vi "ReadSensors.vi"(8 "error in":errorcluster, 11 "UART in":refnum<visa-resource-name>) -> (0 "error out":errorcluster, 2 "Kobuki Sensors  out":T1 {"Charger Source" items=["DISCHARGING"=0, "DOCKING_CHARGED"=2, "DOCKING_CHARGING"=6, "ADAPTER_CHARGED"=18, "ADAPTER_CHARGING"=22]}, 3 "UART out":refnum<visa-resource-name>)   [LabVIEW 2017]
uses:
  KobukiSensors.ctl
  Kobuki Bumps and WheelDrops.ctl
  Kobuki Buttons.ctl
  GetSensorState.ctl
  <vilib>/Instr/_visa.llb/VISA Flush IO Buffer Mask.ctl
  <vilib>/Utility/error.llb/Error Cluster From Error Code.vi
  <vilib>/ErrorRing/Error Ring.xnode
  system/RobotType.ctl
panel:
  out "raw gyro Z":u16(graph)
  out "raw gyro Y":u16(graph)
  out "raw gyro X":u16(graph)
  out "Array":u8[](array[numeric])
  out "Kobuki Sensors 3":T1 {"Charger Source" items=["DISCHARGING"=0, "DOCKING_CHARGED"=2, "DOCKING_CHARGING"=6, "ADAPTER_CHARGED"=18, "ADAPTER_CHARGING"=22]}
  out "Raw Sensors Value 3":u8[][](array[numeric])=[[1, 15, 200, 174, 0, 3, 4, 227, 33, 192, 34, 18, 17, 0, 0, 137, 0, 0], [3, 3, 0, 0, 0, 0, 0, 0, 0, 0, 0, 0, 0, 0, 0, 0, 0, 0], [4, 7, 49, 218, 155, 255, 0, 0, 0, 0, 0, 0, 0, 0, 0, 0, 0, 0], [5, 6, 212, 2, 68, 7, 155, 0, 0, 0, 0, 0, 0, 0, 0, 0, 0, 0], [6, 2, 1, 1, 0, 0, 0, 0, 0, 0, 0, 0, 0, 0, 0, 0, 0, 0], [13, 14, 226, 6, 40, 0, 55, 0, 149, 255, 33, 0, 55, 0, 144, 255, 0, 0], [16, 16, 0, 0, 230, 15, 236, 15, 229, 15, 230, 15, 240, 15, 0, 0, 0, 0]]
  # "Electrical: charging, battery, OI mode"
  # "Sensors: bump, cliff, button, wheel drop"
  # "Motors:"
  # "Inertia"
  # "Electrical: charging, battery, OI mode"
  # "Sensors: bump, cliff, button, wheel drop"
  # "Motors:"
  # "Inertia"
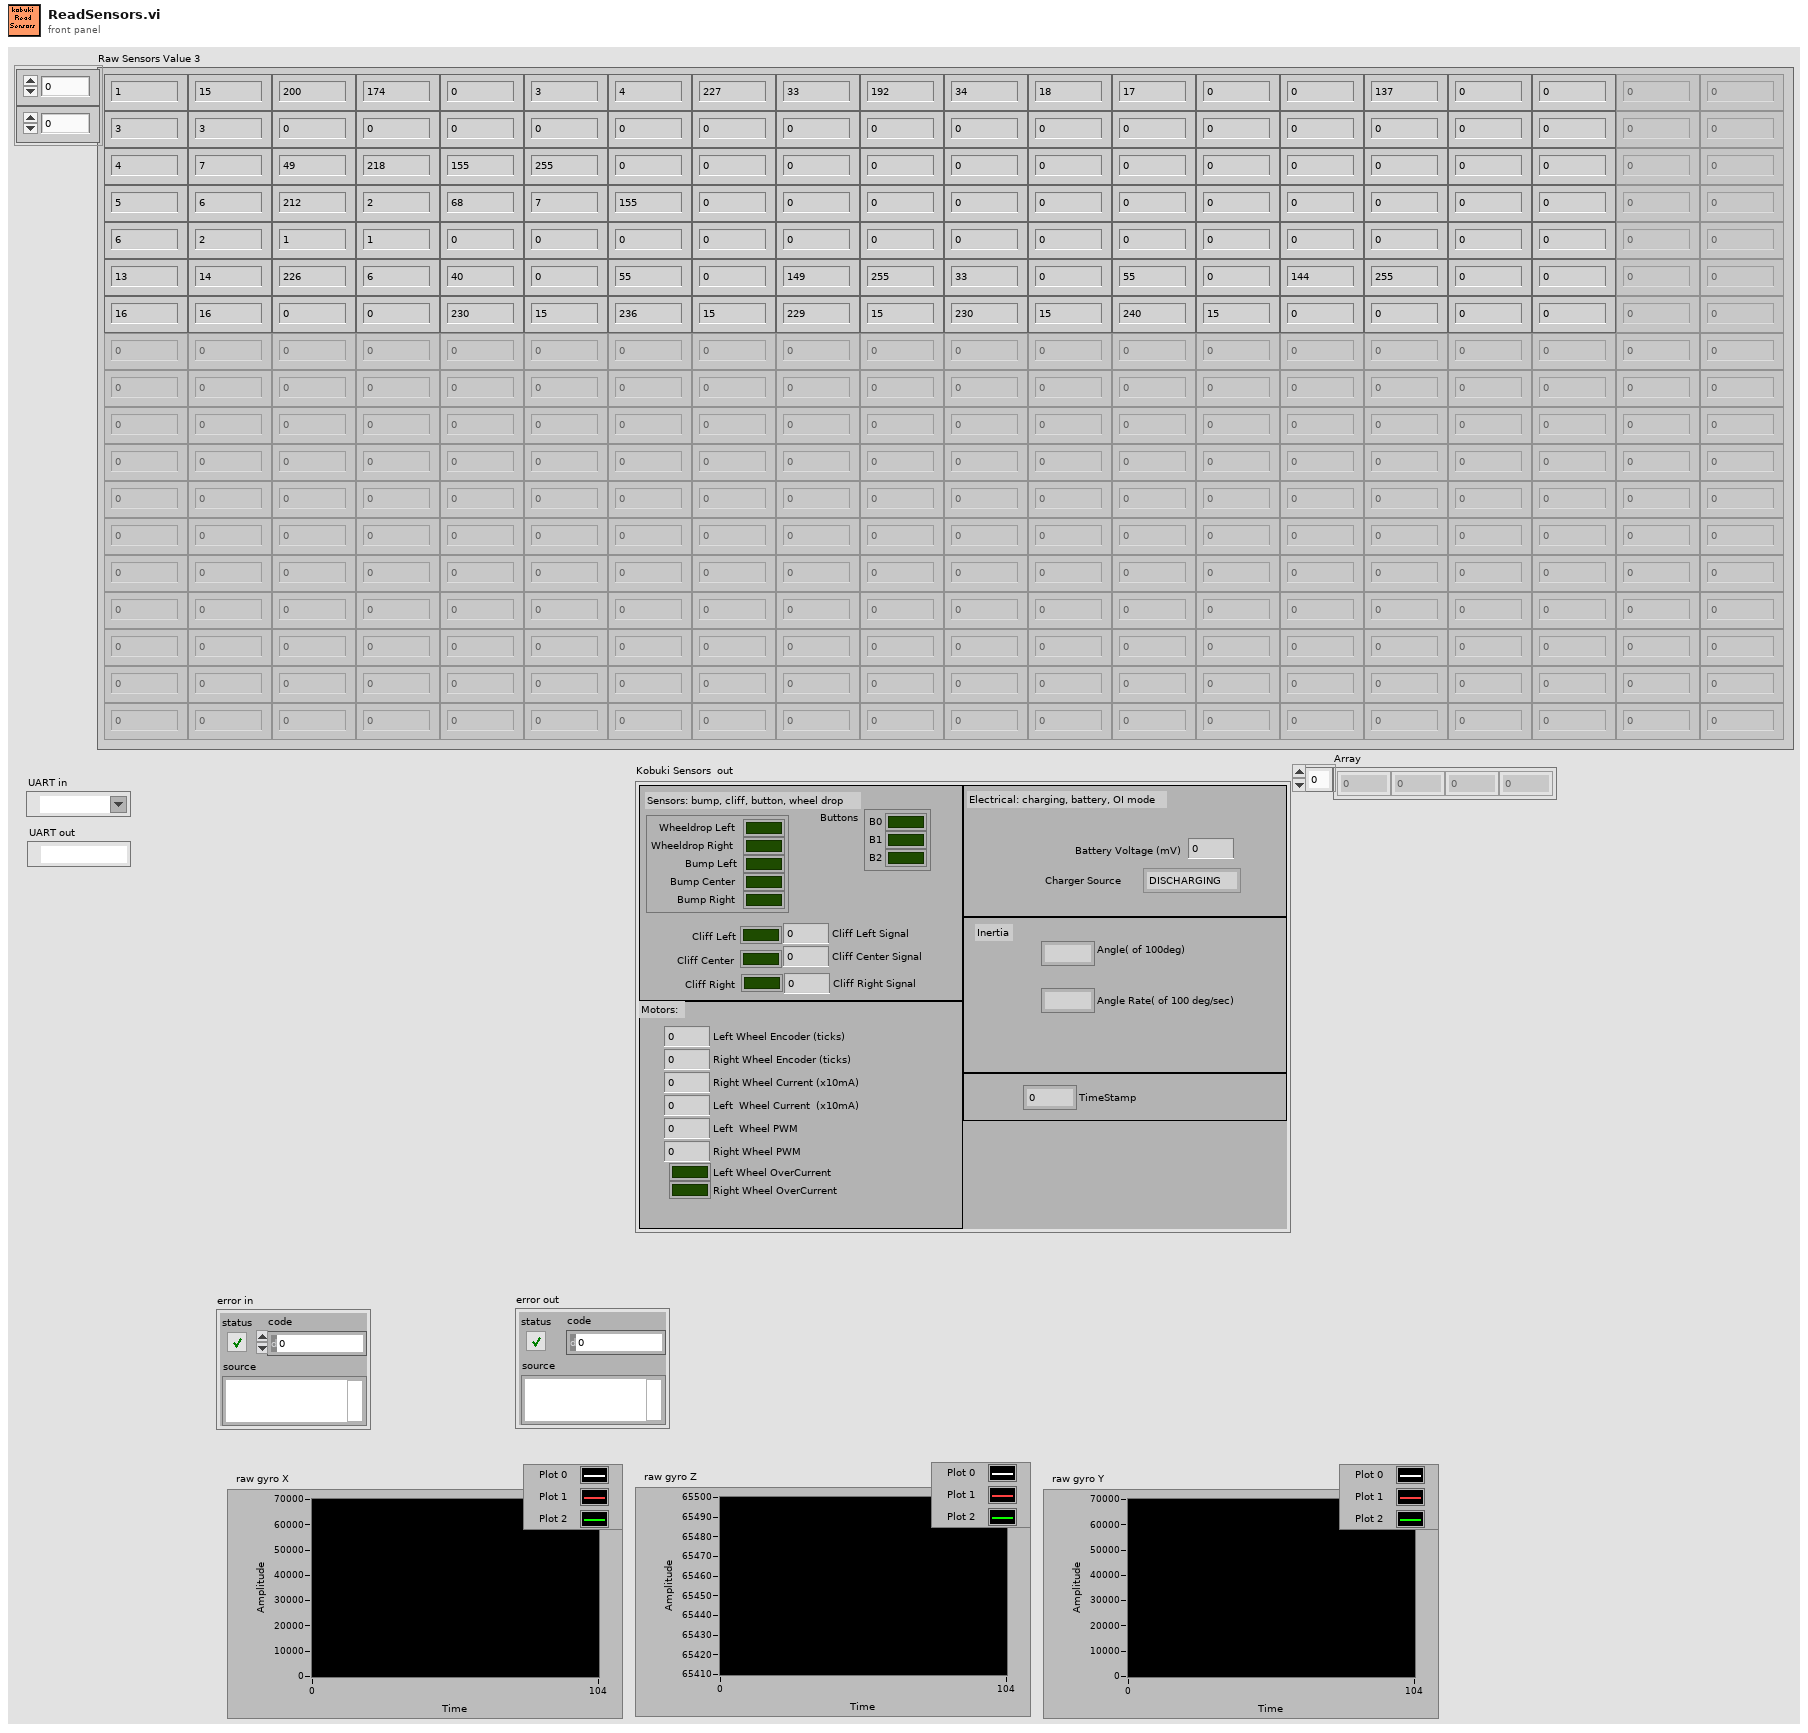
[diagram p1: front panel]
types:
  T1 = typedef "KobukiSensors.ctl" = cluster{"Bumps + Wheel Drops":T2, "Cliff Left":bool, "Cliff Center":bool, "Cliff Right":bool, "Cliff Left Signal":u16, "Cliff Center Signal":u16, "Cliff Right Signal":u16, "Buttons":T3, "Left Wheel Encoder (ticks)":u16, "Right Wheel Encoder (ticks) ":u16, "Left  Wheel PWM":i8, "Right Wheel PWM":i8, "Left Wheel OverCurrent":bool, "Right Wheel OverCurrent ":bool, "Right Wheel Current (x10mA)":i16, "Left  Wheel Current  (x10mA)":i16, "TimeStamp":u16, "Battery Voltage (mV)":i16, "Angle( of 100deg)":i16, "Angle Rate( of 100 deg/sec)":i16, "Charger Source ":i8}
  T2 = typedef "Kobuki Bumps and WheelDrops.ctl" = cluster{"Wheeldrop Left":bool, "Wheeldrop Right":bool, "Bump Left":bool, "Bump Center":bool, "Bump Right":bool}
  T3 = typedef "Kobuki Buttons.ctl" = cluster{"B0":bool, "B1":bool, "B2":bool}
  T4 = typedef "GetSensorState.ctl" = enum16{"GetHeaders", "GetSizeAndPayLoad"}
  T5 = typedef "RobotType.ctl" = enum16{"Kobuki", "iRobot"}
  T6 = typedef "VISA Flush IO Buffer Mask.ctl" = u16
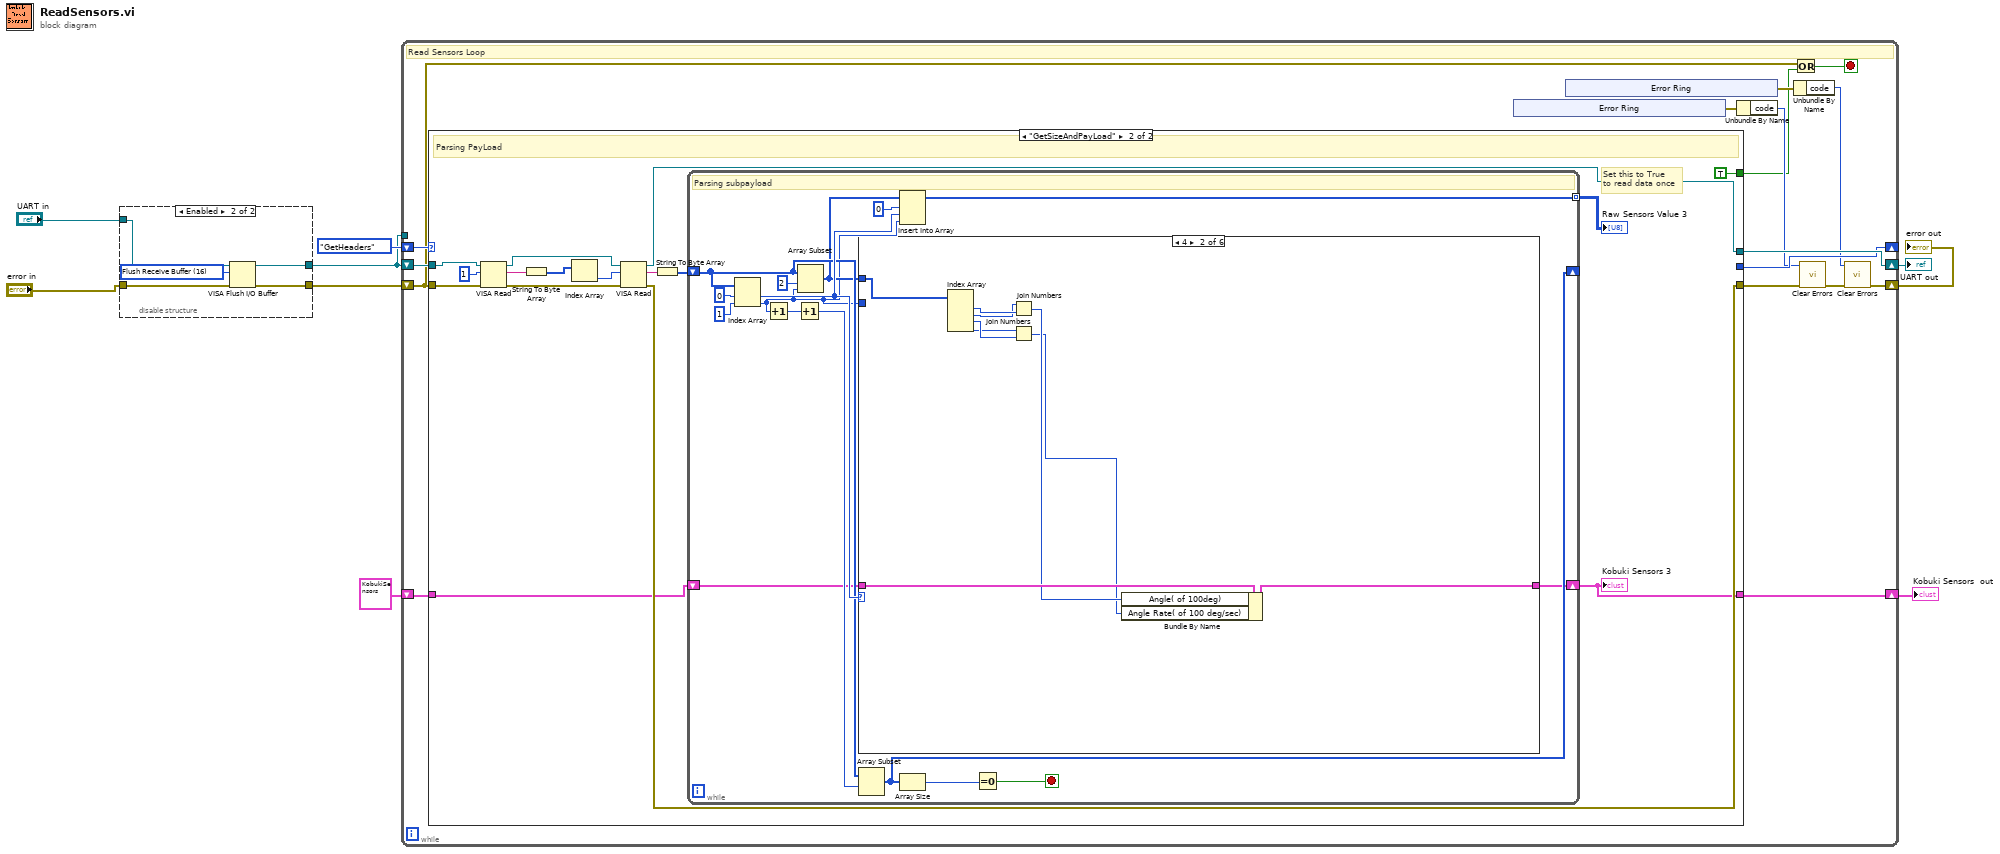
[diagram p0: block diagram]
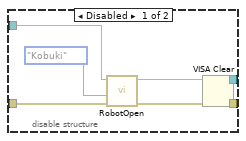
[diagram p2: hidden frame]
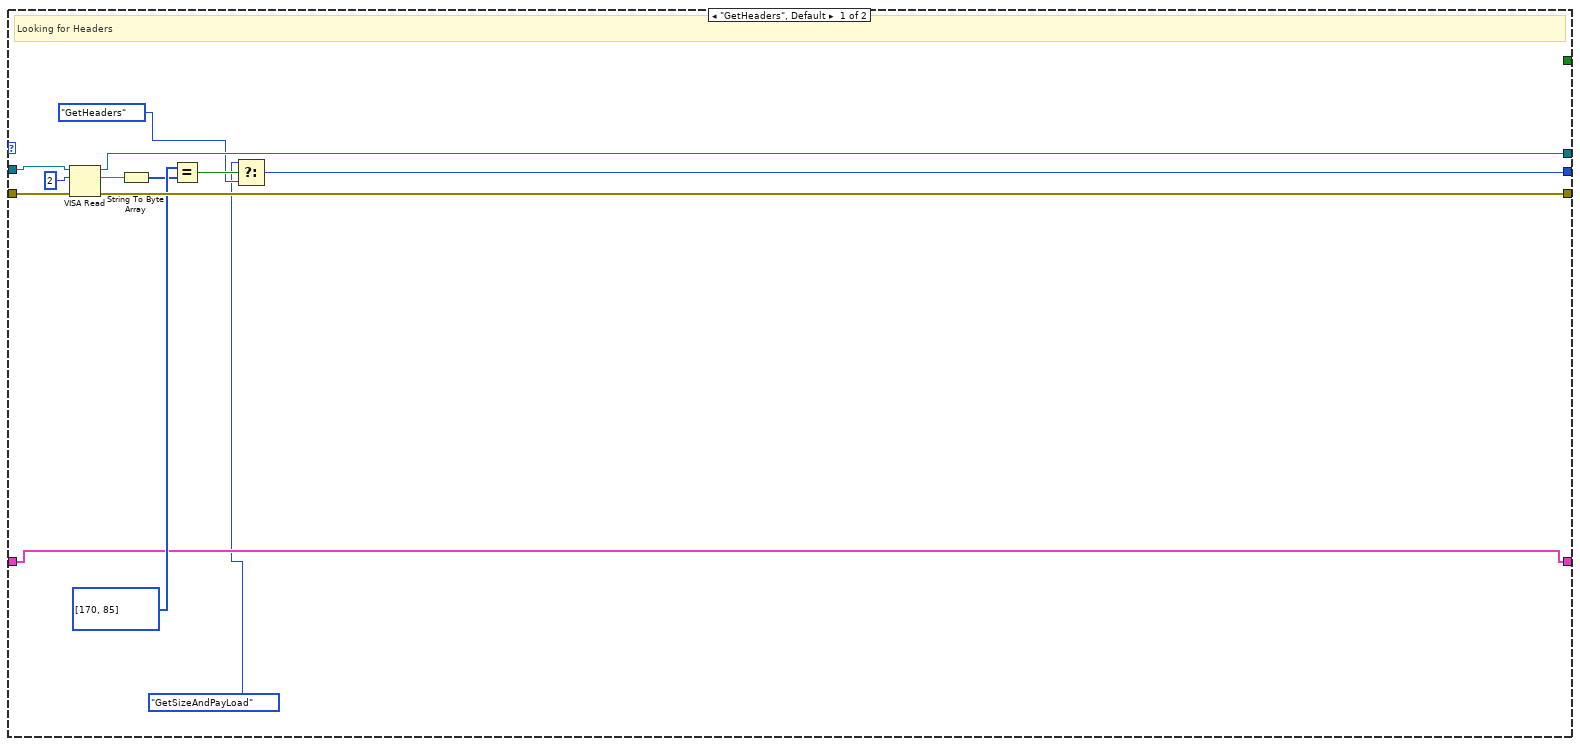
[diagram p3: hidden frame]
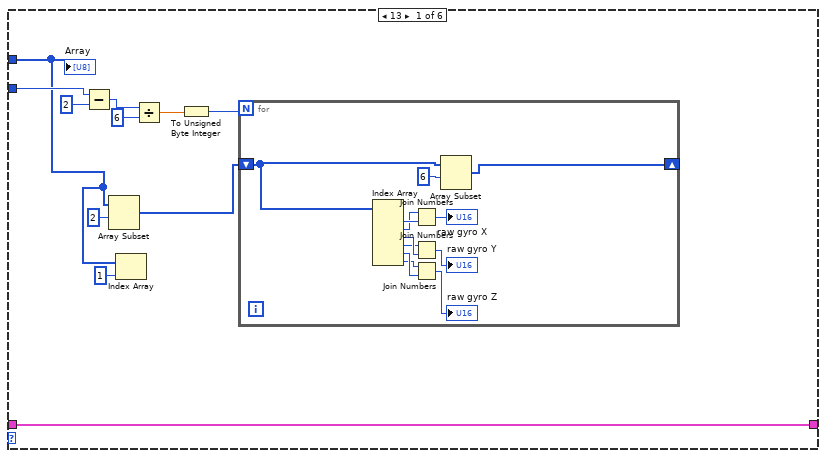
[diagram p4: hidden frame]
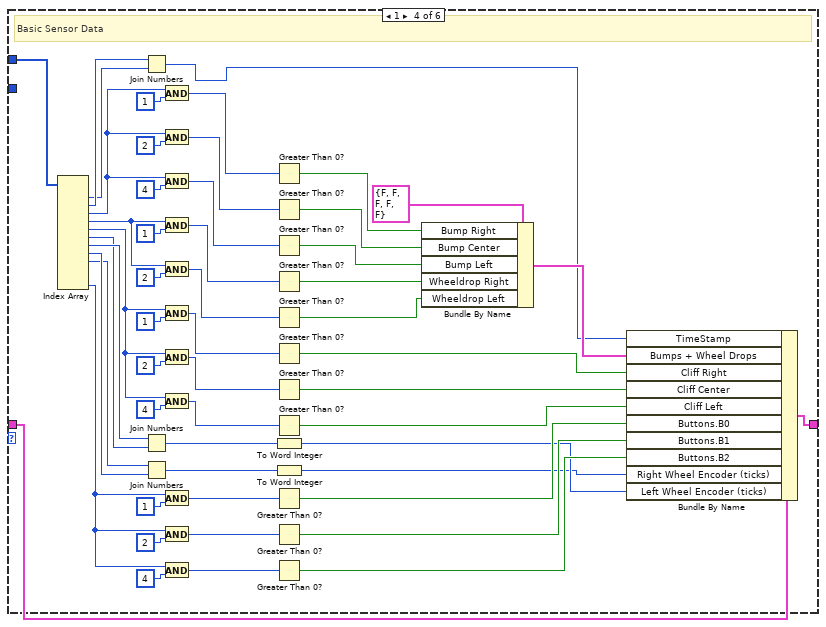
[diagram p6: hidden frame]
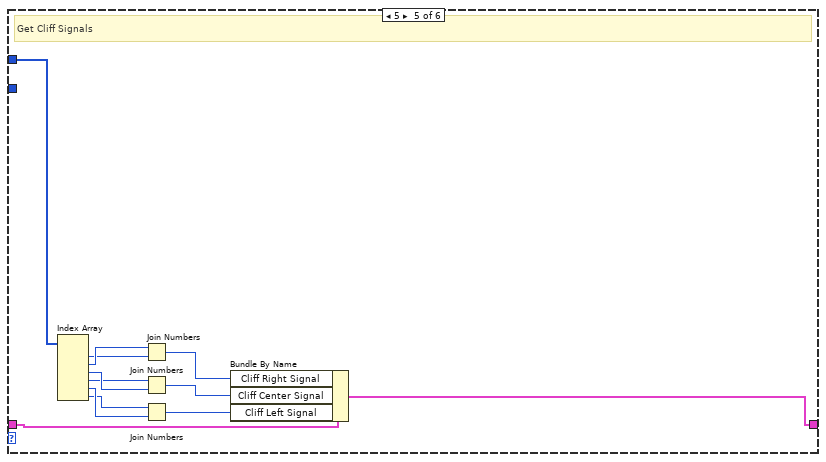
[diagram p7: hidden frame]
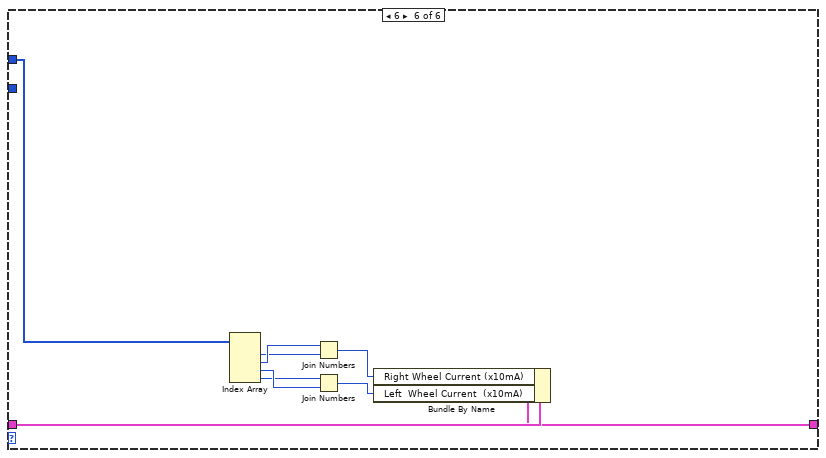
[diagram p8: hidden frame]
diagram:
  n1 = disable-structure shown="Enabled" {
    disable-tunnel: "UART in" -> [w16 w19]
    disable-tunnel: "error in" -> [w15 w20]
    disable-tunnel: [w14 w18] -> w6
    disable-tunnel: [w13 w20] -> w5
    frame Disabled {
      n2 = call "RobotOpen.vi"("error in (no error)"=w15, 9:RobotType."Kobuki" ("RobotType"), "Robot Communication port name"=w16) -> ("error out"=w11:errorcluster, "Robot Communication port name out"=w12:refnum<visa-resource-name>)  [unwired: 7 in]
      n3 = VISA Clear(VISA resource name=w12, error in (no error)=w11) -> (VISA resource name out=w14:refnum<visa-resource-name>, error out=w13:errorcluster)
    }
    frame Enabled {
      w17 = T6 16 items=["Flush Receive Buffer"=16, "Write Transmit Buffer to Device"=32, "Flush Receive Buffer (No I/O)"=64, "Flush Transmit Buffer"=128] ("Mask")
      n4 = VISA Flush I/O Buffer(VISA resource name=w19, mask (16)=w17) -> (VISA resource name out=w18:refnum<visa-resource-name>)  [unwired: 1 in, 1 out]
    }
  }
  n5 = while {
    tunnel: w6 -> [_]
    shift-right: [w28] -> w1
    shift-left: w5 -> [w29]
    shift-right: [w35] -> w2
    shift-left: w6 -> [w36]
    shift-right: [w34] -> _
    shift-left: GetSensorState."GetHeaders" ("Character Count") -> [w33]
    shift-right: [w22] -> w4
    shift-left: T1 {"Bumps + Wheel Drops"={"Wheeldrop Left"=FALSE, "Wheeldrop Right"=FALSE, "Bump Left"=FALSE, "Bump Center"=FALSE, "Bump Right"=FALSE}, "Cliff Left"=FALSE, "Cliff Center"=FALSE, "Cliff Right"=FALSE, "Cliff Left Signal"=0, "Cliff Center Signal"=0, "Cliff Right Signal"=0, "Buttons"={"B0"=FALSE, "B1"=FALSE, "B2"=FALSE}, "Left Wheel Encoder (ticks)"=0, "Right Wheel Encoder (ticks) "=0, "Left  Wheel PWM"=0, "Right Wheel PWM"=0, "Left Wheel OverCurrent"=FALSE, "Right Wheel OverCurrent "=FALSE, "Right Wheel Current (x10mA)"=0, "Left  Wheel Current  (x10mA)"=0, "TimeStamp"=0, "Battery Voltage (mV)"=0, "Angle( of 100deg)"=0, "Angle Rate( of 100 deg/sec)"=0, "Charger Source "=0} ("Kobuki Sensors 2") -> [w21]
    stop <- w32 stop-if-true
    # "Read Sensors Loop"
    n6 = case shown="\"GetSizeAndPayLoad\"" w33 {
      tunnel: w29 -> [w56 w70]
      tunnel: [w55 w67] -> w27
      tunnel: w36 -> [w50 w73]
      tunnel: [w49 w65] -> w35
      tunnel: [w48 _] -> w34
      tunnel: [_ TRUE ("Stop Button 2")] -> w23
      tunnel: [w47 w59] -> w22
      tunnel: w21 -> [w47 w58]
      frame "GetHeaders", Default {
        # "Looking for Headers"
        n7 = VISA Read(VISA resource name=w50, byte count=u32 2 ("Character Count"), error in (no error)=w56) -> (VISA resource name out=w49:refnum<visa-resource-name>, read buffer=w54:string, error out=w55:errorcluster)  [unwired: 1 out]
        n8 = String To Byte Array(string=w54) -> (unsigned byte array=w52:u8[])
        n9 = Equal?(x=u8[] [170, 85] ("unsigned byte array"), y=w52) -> (x = y?=w51:bool)
        n10 = Select(t=GetSensorState."GetSizeAndPayLoad" ("Character Count"), s=w51, f=GetSensorState."GetHeaders" ("Character Count")) -> (s? t:f=w48:T4)
      }
      frame "GetSizeAndPayLoad" {
        # "Set this to True \nto read data once"
        # "Parsing PayLoad"
        n11 = VISA Read(VISA resource name=w73, byte count=u32 1, error in (no error)=w70) -> (VISA resource name out=w69:refnum<visa-resource-name>, read buffer=w71:string, error out=w68:errorcluster)  [unwired: 1 out]
        n12 = String To Byte Array(string=w71) -> (unsigned byte array=w60:u8[])
        n13 = Index Array(array=w60) -> (element=w66:u8)  [unwired: 1 in]
        n14 = VISA Read(VISA resource name=w69, byte count=w66, error in (no error)=w68) -> (VISA resource name out=w65:refnum<visa-resource-name>, read buffer=w64:string, error out=w67:errorcluster)  [unwired: 1 out]
        n15 = String To Byte Array(string=w64) -> (unsigned byte array=w63:u8[])
        n16 = while {
          shift-right: [w82] -> _
          shift-left: w63 -> [w78]
          tunnel: [w85] -> w62 mode=indexing
          shift-right: [w76] -> w59
          shift-left: w58 -> [w75]
          stop <- w80 stop-if-true
          # "Parsing subpayload"
          n17 = Index Array(array=w78, index #1=0 ("index"), index #2=1 ("index")) -> (element #1=w79:u8, element #2=w74:u8)
          n18 = Increment(x=w74) -> (x+1=w83:u8)
          n19 = Increment(x=w83) -> (x+1=w84:u8)
          n20 = Array Subset(array=w78, index=2, length=w74) -> (w77:u8[])
          n21 = case shown="4" w79 {
            tunnel: w77 -> [w92 w121 _ w175 w187 w190]
            tunnel: [w90 w115 w122 w165 w177 w188] -> w76
            tunnel: w75 -> [w90 w116 w122 w132 w176 w189]
            tunnel: w74 -> [w100 _ _ _ _ _]
            frame 13 {
              n22 = Subtract(x=w100, y=u8 2) -> (x-y=w98:u8)
              n23 = Array Subset(array=w92, index=2) -> (w93:u8[])  [unwired: 1 in]
              n24 = Index Array(array=w92, index=1) -> ()  [unwired: 1 out]
              n25 = Divide(x=w98, y=u8 6) -> (x/y=w96:dbl)
              n26 = To Unsigned Byte Integer(number=w96) -> (unsigned 8bit integer=w95:u8)
              n27 = for {
                N: w95 -> [_]
                shift-right: [w111] -> _
                shift-left: w93 -> [w110]
                n28 = Index Array(array=w110) -> (element #1=w109:u8, element #2=w108:u8, element #3=w107:u8, element #4=w106:u8, element #5=w105:u8, element #6=w104:u8)  [unwired: 6 in]
                n29 = Join Numbers(hi=w108, lo=w109) -> ((hi.lo)=→"raw gyro X":u16)
                n30 = Join Numbers(hi=w106, lo=w107) -> ((hi.lo)=→"raw gyro Y":u16)
                n31 = Join Numbers(hi=w104, lo=w105) -> ((hi.lo)=→"raw gyro Z":u16)
                n32 = Array Subset(array=w110, index=6) -> (w111:u8[])  [unwired: 1 in]
              }
              "Array" <- w92
            }
            frame 4 {
              n33 = Index Array(array=w121) -> (element #1=w120:u8, element #2=w119:u8, element #3=w118:u8, element #4=w117:u8)  [unwired: 4 in]
              n34 = Join Numbers(hi=w119, lo=w120) -> ((hi.lo)=w114:u16)
              n35 = Join Numbers(hi=w117, lo=w118) -> ((hi.lo)=w113:u16)
              n36 = Bundle By Name(cluster=w116, "Angle( of 100deg)"=w114, "Angle Rate( of 100 deg/sec)"=w113) -> (w115:T1)
            }
            frame 0, Default {
            }
            frame 1 {
              # "Basic Sensor Data"
              n37 = Index Array(array=w175) -> (element #1=w173:u8, element #2=w174:u8, element #3=w169:u8, element #4=w153:u8, element #5=w147:u8, element #6=w130:u8, element #7=w131:u8, element #8=w127:u8, element #9=w126:u8, element #12=w133:u8)  [unwired: 12 in, 2 out]
              n38 = Join Numbers(hi=w174, lo=w173) -> ((hi.lo)=w123:u16)
              n39 = Join Numbers(hi=w131, lo=w130) -> ((hi.lo)=w129:u16)
              n40 = Join Numbers(hi=w126, lo=w127) -> ((hi.lo)=w125:u16)
              n41 = And(x=w169, y=u8 1 ("element")) -> (x .and. y?=w168:u8)
              n42 = And(x=w169, y=u8 2 ("element")) -> (x .and. y?=w167:u8)
              n43 = And(x=w169, y=u8 4 ("element")) -> (x .and. y?=w166:u8)
              n44 = And(x=w153, y=u8 1 ("element")) -> (x .and. y?=w157:u8)
              n45 = And(x=w153, y=u8 2 ("element")) -> (x .and. y?=w155:u8)
              n46 = And(x=w147, y=u8 1 ("element")) -> (x .and. y?=w150:u8)
              n47 = And(x=w147, y=u8 2 ("element")) -> (x .and. y?=w151:u8)
              n48 = And(x=w147, y=u8 4 ("element")) -> (x .and. y?=w152:u8)
              n49 = And(x=w133, y=u8 1 ("element")) -> (x .and. y?=w139:u8)
              n50 = And(x=w133, y=u8 2 ("element")) -> (x .and. y?=w138:u8)
              n51 = And(x=w133, y=u8 4 ("element")) -> (x .and. y?=w137:u8)
              n52 = Greater Than 0?(x=w168) -> (x > 0?=w163:bool)
              n53 = Greater Than 0?(x=w167) -> (x > 0?=w162:bool)
              n54 = Greater Than 0?(x=w166) -> (x > 0?=w161:bool)
              n55 = Greater Than 0?(x=w157) -> (x > 0?=w156:bool)
              n56 = Greater Than 0?(x=w155) -> (x > 0?=w154:bool)
              n57 = Greater Than 0?(x=w150) -> (x > 0?=w145:bool)
              n58 = Greater Than 0?(x=w151) -> (x > 0?=w144:bool)
              n59 = Greater Than 0?(x=w152) -> (x > 0?=w143:bool)
              n60 = To Word Integer(number=w129) -> (16bit integer=w128:i16)
              n61 = To Word Integer(number=w125) -> (16bit integer=w124:i16)
              n62 = Greater Than 0?(x=w139) -> (x > 0?=w136:bool)
              n63 = Greater Than 0?(x=w138) -> (x > 0?=w135:bool)
              n64 = Greater Than 0?(x=w137) -> (x > 0?=w134:bool)
              n65 = Bundle By Name(cluster=T2 {"Wheeldrop Left"=FALSE, "Wheeldrop Right"=FALSE, "Bump Left"=FALSE, "Bump Center"=FALSE, "Bump Right"=FALSE} ("Bumps + Wheel Drops"), "Bump Right"=w163, "Bump Center"=w162, "Bump Left"=w161, "Wheeldrop Right"=w156, "Wheeldrop Left"=w154) -> (w160:T2)
              n66 = Bundle By Name(cluster=w132, "TimeStamp"=w123, "Bumps + Wheel Drops"=w160, "Cliff Right"=w145, "Cliff Center"=w144, "Cliff Left"=w143, "Buttons.B0"=w136, "Buttons.B1"=w135, "Buttons.B2"=w134, "Right Wheel Encoder (ticks)"=w124, "Left Wheel Encoder (ticks)"=w128) -> (w165:T1)
            }
            frame 5 {
              # "Get Cliff Signals"
              n67 = Index Array(array=w187) -> (element #1=w185:u8, element #2=w186:u8, element #3=w183:u8, element #4=w182:u8, element #5=w180:u8, element #6=w179:u8)  [unwired: 6 in]
              n68 = Join Numbers(hi=w186, lo=w185) -> ((hi.lo)=w184:u16)
              n69 = Join Numbers(hi=w182, lo=w183) -> ((hi.lo)=w181:u16)
              n70 = Join Numbers(hi=w179, lo=w180) -> ((hi.lo)=w178:u16)
              n71 = Bundle By Name(cluster=w176, "Cliff Right Signal"=w184, "Cliff Center Signal"=w181, "Cliff Left Signal"=w178) -> (w177:T1)
            }
            frame 6 {
              n72 = Index Array(array=w190) -> (element #1=w195:u8, element #2=w196:u8, element #3=w193:u8, element #4=w192:u8)  [unwired: 4 in]
              n73 = Join Numbers(hi=w196, lo=w195) -> ((hi.lo)=w194:u16)
              n74 = Join Numbers(hi=w192, lo=w193) -> ((hi.lo)=w191:u16)
              n75 = Bundle By Name(cluster=w189, "Right Wheel Current (x10mA)"=w194, "Left  Wheel Current  (x10mA)"=w191) -> (w188:T1)
            }
          }
          n76 = Array Subset(array=w78, index=w84) -> (w82:u8[])  [unwired: 1 in]
          n77 = Insert Into Array(array=w77, index=0, new element #1=w79, new element #2=w74) -> (w85:u8[])
          n78 = Array Size(array=w82) -> (size(s)=w81:i32)
          n79 = Equal To 0?(x=w81) -> (x = 0?=w80:bool)
        }
        "Raw Sensors Value 3" <- w62
        "Kobuki Sensors 3" <- w59
      }
    }
    n80 = xnode "Error Ring"() -> ("error out"=w25:errorcluster)
    n81 = xnode "Error Ring"() -> ("error out"=w31:errorcluster)
    n82 = Unbundle By Name(w25) -> ("code"=w24:i32)
    n83 = Or(x=w29, y=w23) -> (x .or. y?=w32:bool)
    n84 = Unbundle By Name(w31) -> ("code"=w30:i32)
    n85 = call <vilib>:"Clear Errors.vi"("error in (no error)"=w27, "specific error code to clear (0: all)"=w24) -> ("error out"=w26:errorcluster)  [unwired: 4 in, 1 out]
    n86 = call <vilib>:"Clear Errors.vi"("error in (no error)"=w26, "specific error code to clear (0: all)"=w30) -> ("error out"=w28:errorcluster)  [unwired: 4 in, 1 out]
  }
  "Kobuki Sensors  out" <- w4
  "UART out" <- w2
  "error out" <- w1
